vi "超标浓度设置.vi"(11 "输入":T2) -> (3 "输出":T1)   [LabVIEW 2016, in "德润DR803L超标留样.lvlib"]
uses:
  <vilib>/Utility/miscctls.llb/LVPointTypeDef.ctl
panel:
  in  "汞超标浓度":dbl
  in  "锰超标浓度":dbl
  in  "镍超标浓度":dbl
  in  "锌超标浓度":dbl
  in  "铜超标浓度":dbl
  in  "镉超标浓度":dbl
  in  "铅超标浓度":dbl
  in  "COD超标浓度":dbl
  in  "ORP超标浓度":dbl
  in  "蓝绿藻超标浓度":dbl
  in  "藻密度超标浓度":dbl
  in  "叶绿素a超标浓度":dbl
  in  "浊度超标浓度":dbl
  in  "电导率超标浓度":dbl
  in  "溶解氧超标浓度":dbl
  in  "PH超标浓度":dbl
  in  "取消":bool
  in  "确定":bool
  in  "CODCr超标浓度":dbl
  in  "CODMn超标浓度":dbl
  in  "总氮超标浓度":dbl
  in  "总磷超标浓度":dbl
  in  "氨氮超标浓度":dbl
  # "超标浓度报警配置"
  # "cells/mL"
  # "/"
  # "mg/L"
  # "cells/mL"
  # "mg/L"
  # "mg/L"
  # "/"
  # "μs/cm"
  # "mg/L"
  # "mg/L"
  # "NTU"
  # "mg/L"
  # "μg/L"
  # "mg/L"
  # "mg/L"
  # "mg/L"
  # "mg/L"
  # "mg/L"
  # "mg/L"
  # "mg/L"
  # "mg/L"
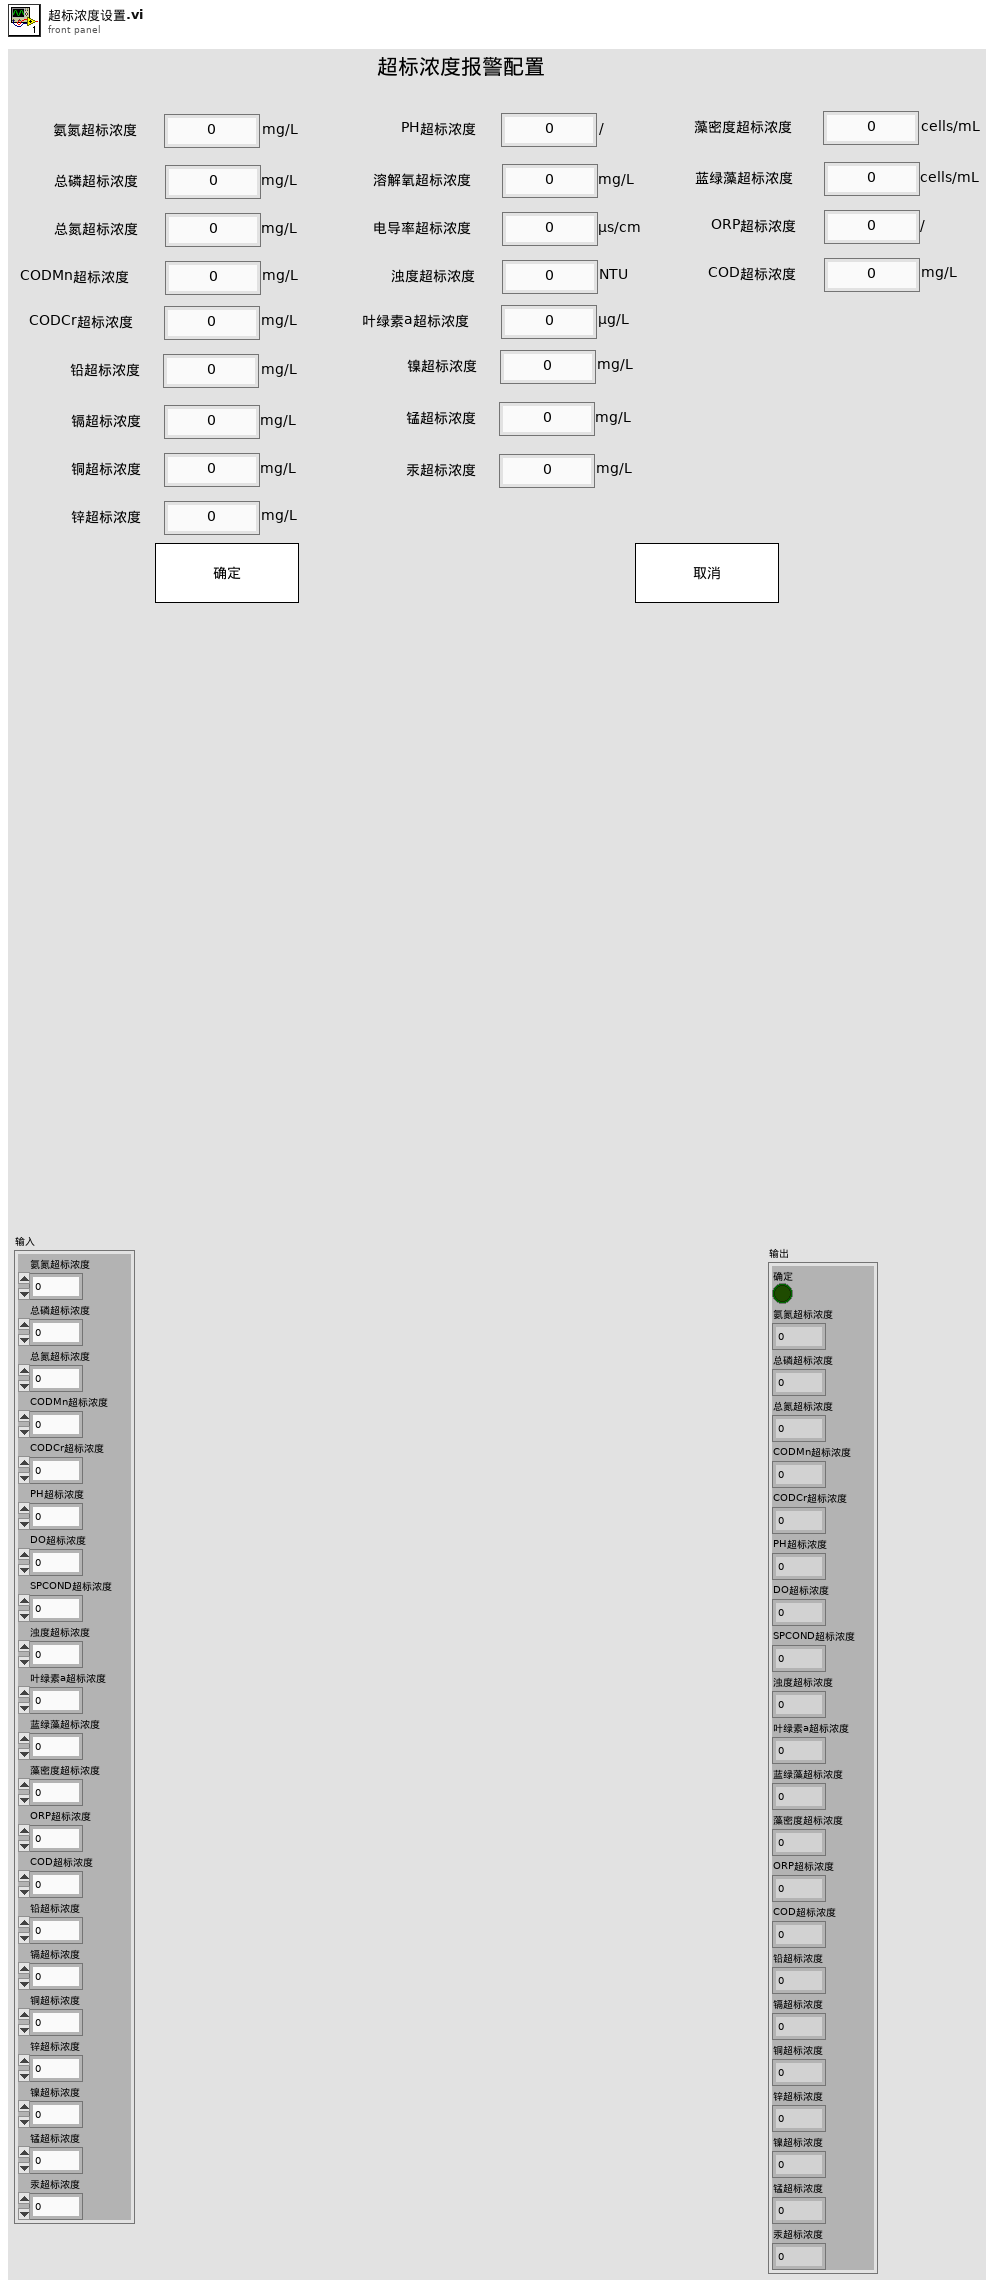
[diagram p1: front panel]
types:
  T1 = cluster{"确定":bool, "氨氮超标浓度":dbl, "总磷超标浓度":dbl, "总氮超标浓度":dbl, "CODMn超标浓度":dbl, "CODCr超标浓度":dbl, "PH超标浓度":dbl, "DO超标浓度":dbl, "SPCOND超标浓度":dbl, "浊度超标浓度":dbl, "叶绿素a超标浓度":dbl, "蓝绿藻超标浓度":dbl, "藻密度超标浓度":dbl, "ORP超标浓度":dbl, "COD超标浓度":dbl, "铅超标浓度":dbl, "镉超标浓度":dbl, "铜超标浓度":dbl, "锌超标浓度":dbl, "镍超标浓度":dbl, "锰超标浓度":dbl, "汞超标浓度":dbl}
  T2 = cluster{"氨氮超标浓度":dbl, "总磷超标浓度":dbl, "总氮超标浓度":dbl, "CODMn超标浓度":dbl, "CODCr超标浓度":dbl, "PH超标浓度":dbl, "DO超标浓度":dbl, "SPCOND超标浓度":dbl, "浊度超标浓度":dbl, "叶绿素a超标浓度":dbl, "蓝绿藻超标浓度":dbl, "藻密度超标浓度":dbl, "ORP超标浓度":dbl, "COD超标浓度":dbl, "铅超标浓度":dbl, "镉超标浓度":dbl, "铜超标浓度":dbl, "锌超标浓度":dbl, "镍超标浓度":dbl, "锰超标浓度":dbl, "汞超标浓度":dbl}
  T3 = typedef "LVPointTypeDef.ctl" = cluster{"Horizontal":i16, "Vertical":i16}
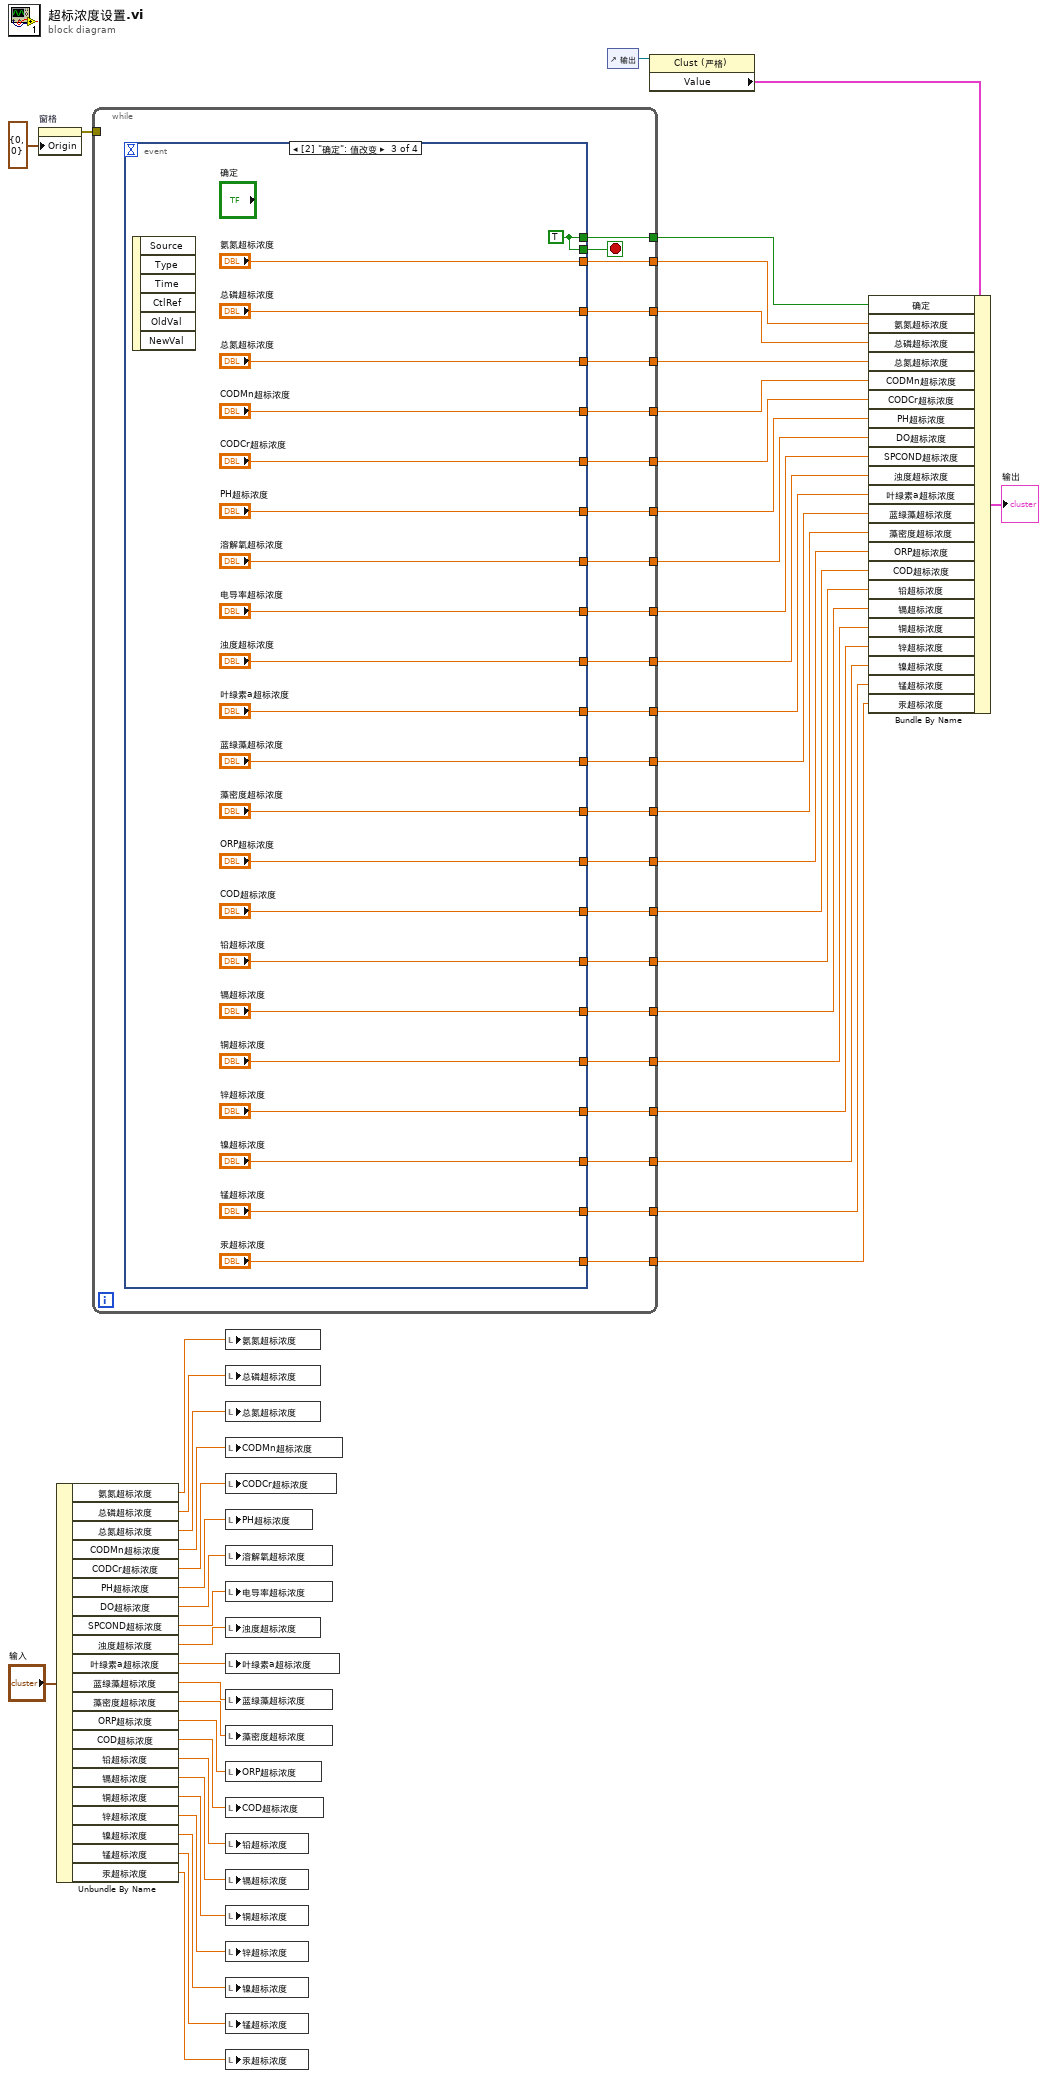
[diagram p0: block diagram]
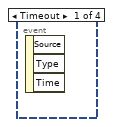
[diagram p2: hidden frame]
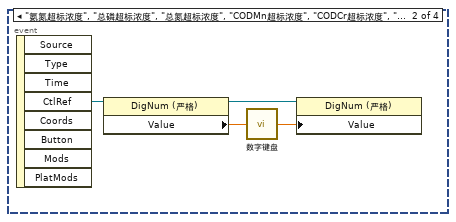
[diagram p3: hidden frame]
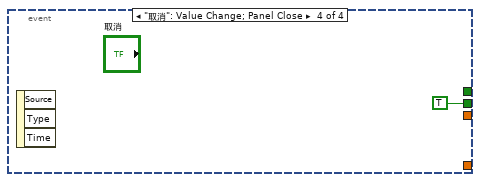
[diagram p4: hidden frame]
diagram:
  n1 = property on="窗格" class="Pane"("Origin"=T3 {"Horizontal"=0, "Vertical"=0} ("原点")) -> (error out=w24:errorcluster)  [unwired: 2 in, 1 out]
  n2 = Unbundle By Name("输入") -> ("氨氮超标浓度"=w41:dbl, "总磷超标浓度"=w40:dbl, "总氮超标浓度"=w39:dbl, "CODMn超标浓度"=w38:dbl, "CODCr超标浓度"=w37:dbl, "PH超标浓度"=w33:dbl, "DO超标浓度"=w32:dbl, "SPCOND超标浓度"=w31:dbl, "浊度超标浓度"=w30:dbl, "叶绿素a超标浓度"=w29:dbl, "蓝绿藻超标浓度"=w28:dbl, "藻密度超标浓度"=w27:dbl, "ORP超标浓度"=w26:dbl, "COD超标浓度"=w25:dbl, "铅超标浓度"=w7:dbl, "镉超标浓度"=w6:dbl, "铜超标浓度"=w5:dbl, "锌超标浓度"=w4:dbl, "镍超标浓度"=w3:dbl, "锰超标浓度"=w2:dbl, "汞超标浓度"=w1:dbl)
  n3 = while {
    tunnel: [w71] -> w48
    tunnel: [w70] -> w47
    tunnel: [w69] -> w46
    tunnel: [w68] -> w45
    tunnel: [w67] -> w44
    tunnel: [w66] -> w43
    tunnel: w24 -> [_]
    tunnel: [w65] -> w23
    tunnel: [w64] -> w22
    tunnel: [w63] -> w21
    tunnel: [w62] -> w20
    tunnel: [w61] -> w19
    tunnel: [w60] -> w18
    tunnel: [w59] -> w17
    tunnel: [w58] -> w16
    tunnel: [w57] -> w15
    tunnel: [w56] -> w14
    tunnel: [w55] -> w13
    tunnel: [w54] -> w12
    tunnel: [w53] -> w11
    tunnel: [w52] -> w10
    tunnel: [w51] -> w9
    tunnel: [w50] -> w8
    stop <- w72 stop-if-true
    n4 = event shown="[2] \"确定\": 值改变" {
      selector: _ -> [_ _ _ _]
      dyn-events: _ -> [_ _ _ _]
      timeout: _ -> [_ _ _ _]
      tunnel: [_ _ w98 TRUE] -> w72
      tunnel: [_ _ w98 _] -> w71
      tunnel: [_ _ "氨氮超标浓度" _] -> w70
      tunnel: [_ _ "总磷超标浓度" _] -> w69
      tunnel: [_ _ "总氮超标浓度" _] -> w68
      tunnel: [_ _ "CODMn超标浓度" _] -> w67
      tunnel: [_ _ "CODCr超标浓度" _] -> w66
      tunnel: [_ _ "PH超标浓度" _] -> w65
      tunnel: [_ _ "溶解氧超标浓度" _] -> w64
      tunnel: [_ _ "电导率超标浓度" _] -> w63
      tunnel: [_ _ "浊度超标浓度" _] -> w62
      tunnel: [_ _ "叶绿素a超标浓度" _] -> w61
      tunnel: [_ _ "蓝绿藻超标浓度" _] -> w60
      tunnel: [_ _ "藻密度超标浓度" _] -> w59
      tunnel: [_ _ "ORP超标浓度" _] -> w58
      tunnel: [_ _ "COD超标浓度" _] -> w57
      tunnel: [_ _ "铅超标浓度" _] -> w56
      tunnel: [_ _ "镉超标浓度" _] -> w55
      tunnel: [_ _ "铜超标浓度" _] -> w54
      tunnel: [_ _ "锌超标浓度" _] -> w53
      tunnel: [_ _ "镍超标浓度" _] -> w52
      tunnel: [_ _ "锰超标浓度" _] -> w51
      tunnel: [_ _ "汞超标浓度" _] -> w50
      event Timeout {
        n5 = event-data() -> ()  [unwired: 1 in, 3 out]
      }
      event "氨氮超标浓度", "总磷超标浓度", "总氮超标浓度", "CODMn超标浓度", "CODCr超标浓度", "PH超标浓度", "溶解氧超标浓度", "电导率超标浓度", "浊度超标浓度", "叶绿素a超标浓度", "藻密度超标浓度", "蓝绿藻超标浓度", "ORP超标浓度", "COD超标浓度", "铅超标浓度", "镉超标浓度", "铜超标浓度", "锌超标浓度", "镍超标浓度", "锰超标浓度", "汞超标浓度": Mouse Down {
        n6 = event-data() -> ("CtlRef"=w76:refnum<vi>)  [unwired: 1 in, 7 out]
        n7 = property class="DigNum (严格)"(reference=w76) -> (reference out=w74:refnum<vi>, "Value"=w75:dbl)  [unwired: 1 in, 1 out]
        n8 = call "数字键盘.vi"("OldNumber"=w75) -> ("NewNumber"=w73:sgl)
        n9 = property class="DigNum (严格)"(reference=w74, "Value"=w73) -> ()  [unwired: 1 in, 2 out]
      }
      event "确定": Value Change {
        w98 = TRUE
        n10 = event-data() -> ()  [unwired: 1 in, 6 out]
      }
      event "取消": Value Change; Panel Close {
        n11 = event-data() -> ()  [unwired: 1 in, 3 out]
      }
    }
  }
  n12 = local write "氨氮超标浓度"(w41) -> ()
  n13 = local write "总磷超标浓度"(w40) -> ()
  n14 = local write "总氮超标浓度"(w39) -> ()
  n15 = local write "CODMn超标浓度"(w38) -> ()
  n16 = local write "CODCr超标浓度"(w37) -> ()
  n17 = local write "PH超标浓度"(w33) -> ()
  n18 = local write "溶解氧超标浓度"(w32) -> ()
  n19 = local write "电导率超标浓度"(w31) -> ()
  n20 = local write "浊度超标浓度"(w30) -> ()
  n21 = local write "叶绿素a超标浓度"(w29) -> ()
  n22 = local write "蓝绿藻超标浓度"(w28) -> ()
  n23 = local write "藻密度超标浓度"(w27) -> ()
  n24 = local write "ORP超标浓度"(w26) -> ()
  n25 = local write "COD超标浓度"(w25) -> ()
  n26 = local write "铅超标浓度"(w7) -> ()
  n27 = local write "镉超标浓度"(w6) -> ()
  n28 = local write "铜超标浓度"(w5) -> ()
  n29 = local write "锌超标浓度"(w4) -> ()
  n30 = local write "镍超标浓度"(w3) -> ()
  n31 = local write "锰超标浓度"(w2) -> ()
  n32 = local write "汞超标浓度"(w1) -> ()
  n33 = control-ref of="输出"() -> (w34:refnum<vi>)
  n34 = property class="Clust (严格)"(reference=w34) -> ("Value"=w49:T1)  [unwired: 1 in, 2 out]
  n35 = Bundle By Name(cluster=w49, "确定"=w48, "氨氮超标浓度"=w47, "总磷超标浓度"=w46, "总氮超标浓度"=w45, "CODMn超标浓度"=w44, "CODCr超标浓度"=w43, "PH超标浓度"=w23, "DO超标浓度"=w22, "SPCOND超标浓度"=w21, "浊度超标浓度"=w20, "叶绿素a超标浓度"=w19, "蓝绿藻超标浓度"=w18, "藻密度超标浓度"=w17, "ORP超标浓度"=w16, "COD超标浓度"=w15, "铅超标浓度"=w14, "镉超标浓度"=w13, "铜超标浓度"=w12, "锌超标浓度"=w11, "镍超标浓度"=w10, "锰超标浓度"=w9, "汞超标浓度"=w8) -> (→"输出":T1)
